vi "6 motor arcade drive.vi"(8 "Y Axis":dbl, 11 "X Axis":dbl) -> ()   [LabVIEW 2017]
uses:
  <vilib>/Rock Robotics/Network Tables/NT Write Number.vi
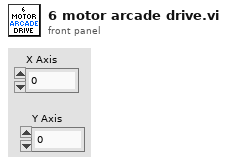
[diagram p1: front panel]
types:
  T1 = typedef "WPI_MotorControlDeviceRef.ctl" = cluster{"DeviceStatus":errorcluster, "Type":T2, "PWM":cluster{"PWM Channel":T3, "DeadBand":T4}, "CAN":cluster{"Device Number":u8, "SetOutput VI Ref":variant, "GetOutput VI Ref":variant, "Enable VI Ref":variant, "Disable VI Ref":variant, "Data":variant}, "Invert":bool, "DIO PWM":cluster{"PWM \"Enable\" Channel":T3, "DIOChannel":T5, "PWM Rate":dbl}}
  T2 = typedef "WPI_MotorControlType.ctl" = enum16{"PWM", "CAN", "DIO PWM"}
  T3 = typedef "FPGA_DIOPWMChannel.ctl" = enum8{"PWM 0", "PWM 1", "PWM 2", "PWM 3", "PWM 4", "PWM 5", "PWM 6", "PWM 7", "PWM 8", "PWM 9", "PWM MXP 0", "PWM MXP 1", "PWM MXP 2", "PWM MXP 3", "PWM MXP 4", "PWM MXP 5", "PWM MXP 6", "PWM MXP 7", "PWM MXP 8", "PWM MXP 9", "Invalid"}
  T4 = typedef "WPI_PWMDeadband.ctl" = cluster{"Name":string, "maxPositivePwm":i32, "minPositivePwm":i32, "centerPwm":i32, "maxNegativePwm":i32, "minNegativePwm":i32, "angularRange":u16}
  T5 = typedef "FPGA_DIOChannel.ctl" = enum8{"DIO 0", "DIO 1", "DIO 2", "DIO 3", "DIO 4", "DIO 5", "DIO 6", "DIO 7", "DIO 8", "DIO 9", "DIO MXP 0", "DIO MXP 1", "DIO MXP 2", "DIO MXP 3", "DIO MXP 4", "DIO MXP 5", "DIO MXP 6", "DIO MXP 7", "DIO MXP 8", "DIO MXP 9", "DIO MXP 10", "DIO MXP 11", "DIO MXP 12", "DIO MXP 13", "DIO MXP 14", "DIO MXP 15", "SPI Port CS1", "SPI Port CS2", "SPI Port CS3", "SPI Port MISO", "SPI Port MOSI", "Invalid"}
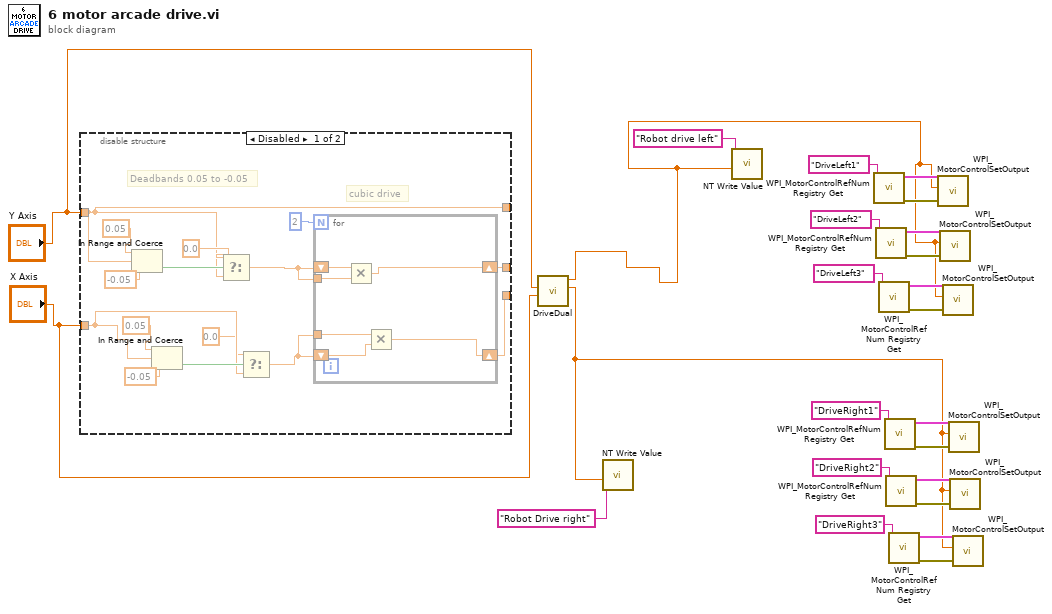
[diagram p0: block diagram]
diagram:
  n1 = disable-structure shown="Disabled" {
    disable-tunnel: "X Axis" -> [w30 _]
    disable-tunnel: "Y Axis" -> [w25 _]
    disable-tunnel: [w27 _] -> _
    disable-tunnel: [w26 _] -> _
    disable-tunnel: [w25 _] -> _
    frame Disabled {
      # "cubic drive"
      # "Deadbands 0.05 to -0.05"
      n2 = In Range and Coerce(upper limit=0.05, x=w25, lower limit=-0.05) -> (In Range?=w39:bool)  [unwired: 1 out]
      n3 = In Range and Coerce(upper limit=0.05, x=w30, lower limit=-0.05) -> (In Range?=w34:bool)  [unwired: 1 out]
      n4 = Select(t=0.0, s=w39, f=w25) -> (s? t:f=w32:dbl)
      n5 = Select(t=0.0, s=w34, f=w30) -> (s? t:f=w31:dbl)
      n6 = for {
        N: 2 -> [_]
        shift-right: [w40] -> w27
        shift-left: w32 -> [w45]
        shift-right: [w41] -> w26
        shift-left: w31 -> [w43]
        tunnel: w32 -> [w44]
        tunnel: w31 -> [w42]
        n7 = Multiply(x=w45, y=w44) -> (x*y=w40:dbl)
        n8 = Multiply(x=w42, y=w43) -> (x*y=w41:dbl)
      }
    }
    frame Enabled {
    }
  }
  n9 = call "DriveDual.vi"("YAxis"="X Axis", "XAxis"="Y Axis") -> ("Right"=w3:dbl, "Left"=w4:dbl)  [unwired: 8 in]
  n10 = call-poly <vilib>:"NT Write Value.vi"("Numeric"=w3, "Name"="Robot Drive right") -> ()  [unwired: 9 in, 1 out]
  n11 = call-poly <vilib>:"NT Write Value.vi"("Numeric"=w4, "Name"="Robot drive left") -> ()  [unwired: 9 in, 1 out]
  n12 = call <vilib>:"WPI_MotorControlRefNum Registry Get.vi"("refnum name"="DriveLeft1") -> ("error out"=w22:errorcluster, "MotorControlDevRef"=w21:T1)  [unwired: 9 in]
  n13 = call <vilib>:"WPI_MotorControlRefNum Registry Get.vi"("refnum name"="DriveLeft2") -> ("error out"=w17:errorcluster, "MotorControlDevRef"=w18:T1)  [unwired: 9 in]
  n14 = call <vilib>:"WPI_MotorControlRefNum Registry Get.vi"("refnum name"="DriveLeft3") -> ("error out"=w16:errorcluster, "MotorControlDevRef"=w15:T1)  [unwired: 9 in]
  n15 = call <vilib>:"WPI_MotorControlRefNum Registry Get.vi"("refnum name"="DriveRight1") -> ("error out"=w11:errorcluster, "MotorControlDevRef"=w12:T1)  [unwired: 9 in]
  n16 = call <vilib>:"WPI_MotorControlRefNum Registry Get.vi"("refnum name"="DriveRight2") -> ("error out"=w10:errorcluster, "MotorControlDevRef"=w9:T1)  [unwired: 9 in]
  n17 = call <vilib>:"WPI_MotorControlRefNum Registry Get.vi"("refnum name"="DriveRight3") -> ("error out"=w5:errorcluster, "MotorControlDevRef"=w6:T1)  [unwired: 9 in]
  n18 = call <vilib>:"WPI_MotorControlSetOutput.vi"("error in (no error)"=w22, "Output"=w4, "MotorControlDevRef"=w21) -> ()  [unwired: 6 in, 3 out]
  n19 = call <vilib>:"WPI_MotorControlSetOutput.vi"("error in (no error)"=w17, "Output"=w4, "MotorControlDevRef"=w18) -> ()  [unwired: 6 in, 3 out]
  n20 = call <vilib>:"WPI_MotorControlSetOutput.vi"("error in (no error)"=w16, "Output"=w4, "MotorControlDevRef"=w15) -> ()  [unwired: 6 in, 3 out]
  n21 = call <vilib>:"WPI_MotorControlSetOutput.vi"("error in (no error)"=w11, "Output"=w3, "MotorControlDevRef"=w12) -> ()  [unwired: 6 in, 3 out]
  n22 = call <vilib>:"WPI_MotorControlSetOutput.vi"("error in (no error)"=w10, "Output"=w3, "MotorControlDevRef"=w9) -> ()  [unwired: 6 in, 3 out]
  n23 = call <vilib>:"WPI_MotorControlSetOutput.vi"("error in (no error)"=w5, "Output"=w3, "MotorControlDevRef"=w6) -> ()  [unwired: 6 in, 3 out]
